vi "DAQX mod 1SDI v00.vi"(0 "resource name":refnum<k15>="PXI1Slot2", 1 "close (T)":bool=TRUE, 2 "Record Data":bool, 3 "numSamples":i32=-1, 4 "max time (s)":dbl=10.0 caption="max time", 5 "min sample rate":dbl=100000000.0, 6 "File location":path, 7 "error in":errorcluster, 8 "reference position":dbl=50.0, 9 "IIR filter specifications":T1={"Topology"=enum."Butterworth", "Type"=enum."Lowpass", "Order"=1, "Lower Fc"=100.0, "Upper Fc"=200.0, "PB Ripple"=1.0, "SB Attenuation"=60.0} {"PB Ripple" format="%0.2f"; "SB Attenuation" format="%0.2f"; "Lower Fc" format="%0.2p"; "Upper Fc" format="%0.2p"}, 10 "Type of\nmeasurement":u16, 11 "Name root":string, 12 "File Name":path=path "C:/Documents and Settings/QIM/My Documents/LabVIEW Data/111016-discord-gain9-seed40-3/ele-0000mV-d0150mV-g9-s40.lvm", 13 "channel parameters":T3(array[cluster])=[{"channel name"="0", "input impedance"=0, "maximum input frequency"=30000000.0, "vertical coupling"=1, "probe attenuation"=1.0, "vertical range"=2.0, "vertical offset"=0.0, "channel enabled"=TRUE}, {"channel name"="1", "input impedance"=0, "maximum input frequency"=30000000.0, "vertical coupling"=1, "probe attenuation"=1.0, "vertical range"=2.0, "vertical offset"=0.0, "channel enabled"=TRUE}] {"input impedance" items=["1 mega ohm"=0, "50 ohms"=2]; "vertical coupling" items=["AC", "DC", "Ground"]}, 14 "Shot noise start":bool, 15 "reset sn":bool) -> (16 "Signal 1":dbl[](graph), 17 "conditional variance":dbl, 18 "error out TDMS":errorcluster caption="error out", 19 "covariance":dbl, 20 "Variance 2 normalised to SNL":dbl(graph), 21 "Signal 2":dbl[](graph), 22 "Parameters values file":string, 23 "Variance 1 normalised to SNL":dbl(graph), 24 "actualSamples 0":i32, 26 "actualSamples 1":i32, 27 "error out":errorcluster caption="error out final")   [LabVIEW 2013]
doc: "Configures and acquires data from an NI-SCOPE high-speed digitizer.\n--------------------\n\nThis Express VI is configured as follows:\n\nDevice: PXI1Slot2 (PXI-5122)\nSample Rate (S/s): 100M\nRecord length: 2k\nAcquisition Mode: N Samples\nChannel 0\n - Range (V): 2\n - Offset (V): 0\n - Probe attenuation: 1\n - Coupling: \n - Input impedence: 1 \n - Bandwidth (Hz): 0\nChannel 1\n - Range (V): 2\n - Offset (V): 0\n - Probe attenuation: 1\n - Coupling: \n - Input impedence: 1 \n - Bandwidth (Hz): 0\nImmediate"
uses:
  <instrlib>/niScope/Controls/niScope vertical coupling.ctl
  <instrlib>/niScope/Controls/niScope timestamp type.ctl
  <vilib>/Analysis/5stat.llb/RMS (DBL).vi
  <vilib>/Analysis/baseanly.llb/Mean (DBL).vi
  <instrlib>/niScope/Acquire/Fetch/niScope Multi Fetch Binary 16.vi
  <instrlib>/niScope/Acquire/Fetch/niScope Multi Fetch WDT.vi
  <vilib>/measure/macond.llb/IIR Filter for N Chan.vi
  Global VIs/shotnoise.vi
  <instrlib>/niScope/Configure/Trigger/niScope Configure Trigger Immediate.vi
  <vilib>/measure/NI_MAPro.lvlib
  <vilib>/Analysis/NI_AALPro.lvlib
  <vilib>/Analysis/NI_AALBase.lvlib
panel:
  out "gain 1":dbl
  out "offset 1":dbl
  out "xIncrement 1":dbl
  out "relativeInitialX 1":dbl
  out "file location into parameter files":path
  out "size(s)":i32
  out "gain 0":dbl
  out "offset 0":dbl
  out "xIncrement 0":dbl
  out "relativeInitialX 0":dbl
  out "actual sample rate":dbl
  in  "Additional text":string
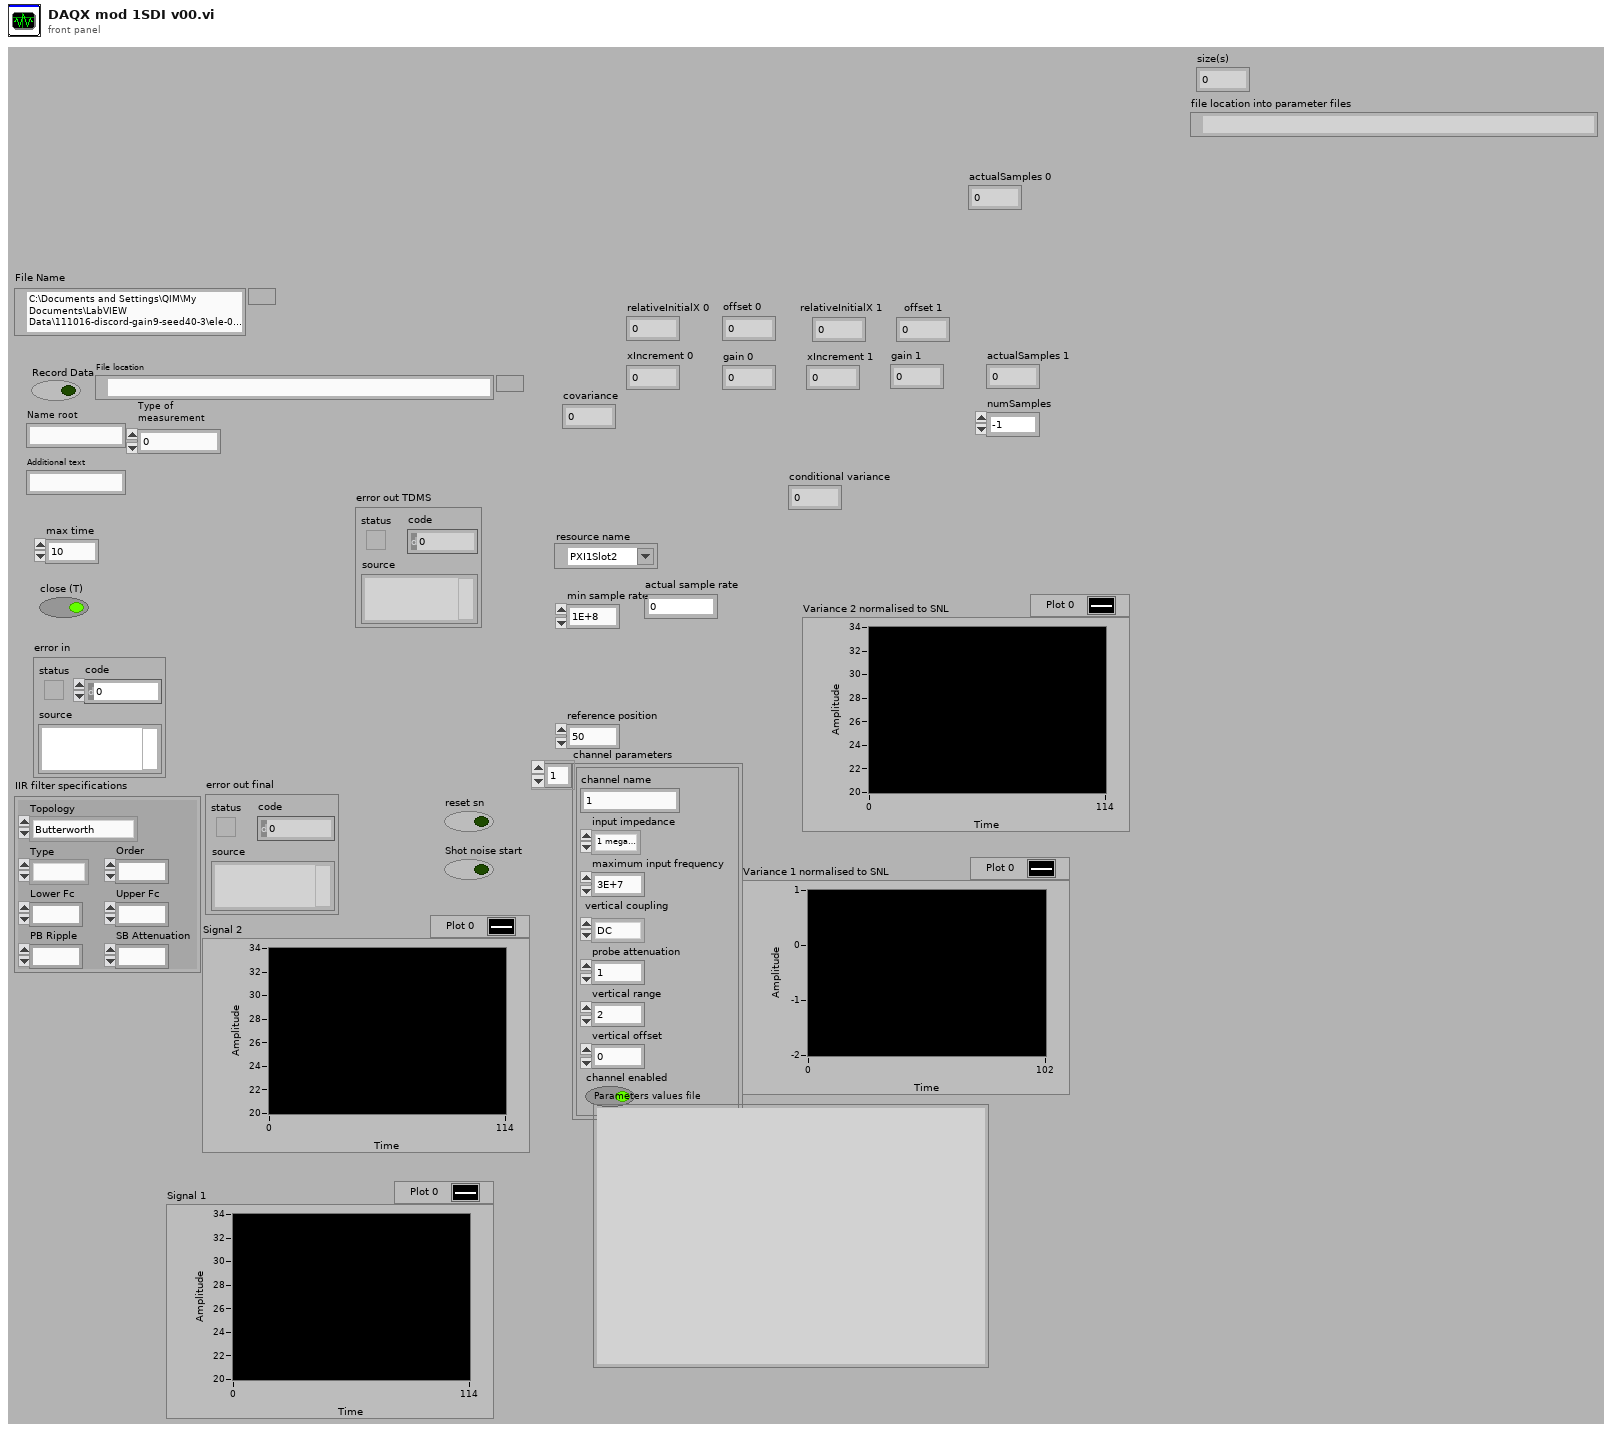
[diagram p1: front panel]
types:
  T1 = cluster{"Topology":enum16{"Off", "Butterworth", "Chebyshev", "Inverse Chebyshev", "Elliptic", "Bessel"}, "Type":enum16{"Lowpass", "Highpass", "Bandpass", "Bandstop"}, "Order":i32, "Lower Fc":dbl, "Upper Fc":dbl, "PB Ripple":dbl, "SB Attenuation":dbl}
  T2 = typedef "niScope vertical coupling.ctl" = i32
  T3 = cluster{"channel name":string, "input impedance":u32, "maximum input frequency":dbl, "vertical coupling":T2, "probe attenuation":dbl, "vertical range":dbl, "vertical offset":dbl, "channel enabled":bool}[]
  T4 = typedef "niScope timestamp type.ctl" = i32
  T5 = cluster{"actualSamples":i32, "absoluteInitialX":dbl, "relativeInitialX":dbl, "xIncrement":dbl, "offset":dbl, "gain":dbl, "reserved1":dbl, "reserved2":dbl}[]
  T6 = cluster{"actualSamples":i32, "absoluteInitialX":dbl, "relativeInitialX":dbl, "xIncrement":dbl, "offset":dbl, "gain":dbl, "reserved1":dbl, "reserved2":dbl}
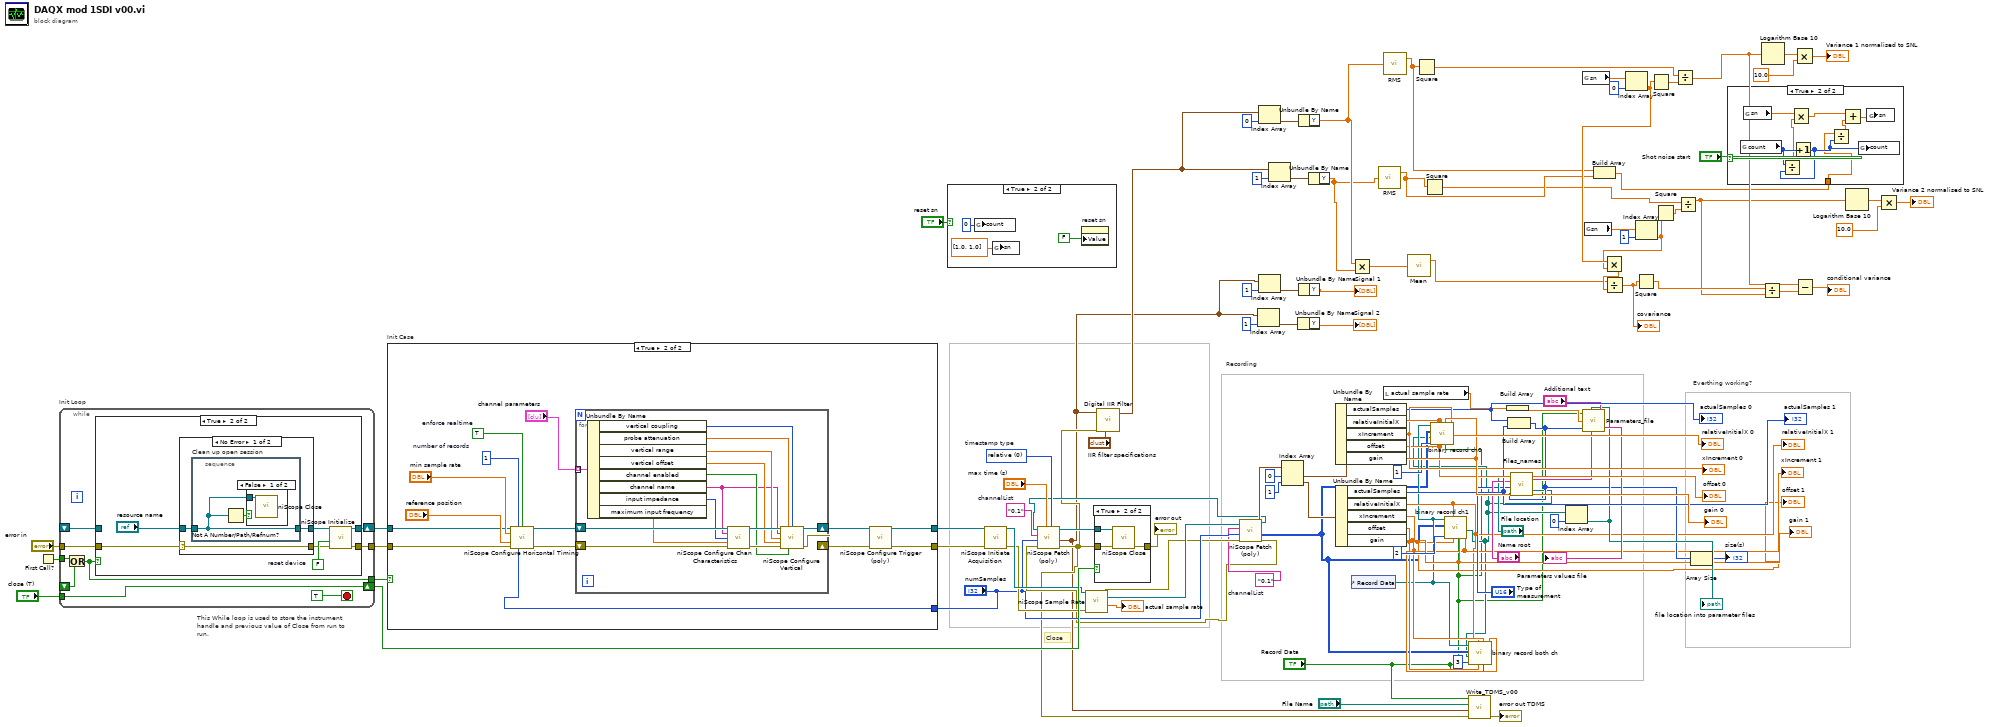
[diagram p0: block diagram]
diagram:
  w25 = "0,1"  # channelList
  w100 = T4 0 items=["relative", "absolute"]  # timestamp type
  w103 = "0,1"  # channelList
  # "Everthing working?"
  # "Recording"
  # "This While loop is used to store the instrument handle and previous value of Close from run to run."
  # "Close"
  n1 = First Call?() -> (First Call?: T/F=w99:bool)
  n2 = while "Init Loop" {
    tunnel: w99 -> [w114]
    shift-right: [w113] -> w95
    shift-left: _ -> [w110]
    tunnel: "close (T)" -> [w113]
    shift-right: [w112] -> w98
    shift-left: _ -> [w111]
    tunnel: [w108] -> w97
    tunnel: "error in" -> [w107]
    tunnel: [w106] -> w96
    stop <- TRUE ("stopInit") stop-if-true
    n3 = Or(x=w114, y=w110) -> (x .or. y?=w106:bool)
    n4 = case "Select_Init" shown="True" w106 {
      tunnel: [w116 w121] -> w112
      tunnel: w111 -> [w116 _]
      tunnel: [w115 w120] -> w108
      tunnel: w107 -> [w115 w119]
      frame False {
      }
      frame True {
        w122 = FALSE  # reset device
        n5 = case shown="No Error" w119 {
          selector: w119 -> [w124 w130]
          tunnel: [w126 w131] -> w123
          tunnel: "resource name" -> [w125 w131]
          tunnel: [w124 w130] -> w118
          frame No Error {
            n6 = stacked-sequence "Clean up open session" {
              tunnel: w125 -> [w127]
              tunnel: [w127] -> w126
              frame #0 {
                n7 = Not A Number/Path/Refnum?(number/path/refnum=w127) -> (NaN/Path/Refnum?=w128:bool)
                n8 = case shown="False" w128 {
                  tunnel: w127 -> [w129 _]
                  frame False {
                    n9 = call <instrlib>:"niScope Close.vi"("instrument handle"=w129) -> ()  [unwired: 1 in, 14 out]
                  }
                  frame True {
                  }
                }
              }
            }
          }
          frame Error {
          }
        }
        n10 = call <instrlib>:"niScope Initialize.vi"("resource name"=w123, "reset device"=w122, "error in"=w118) -> ("instrument handle"=w121:refnum<k15>, "error out"=w120:errorcluster)  [unwired: 2 in, 9 out]
      }
    }
  }
  n11 = case "Init Case" shown="True" w96 {
    tunnel: w97 -> [w132 w138]
    tunnel: [w132 w140] -> w102
    tunnel: [w133 w141] -> w101
    tunnel: w98 -> [w133 w139]
    tunnel: "numSamples" -> [_ w134]
    frame False {
    }
    frame True {
      w146 = 1  # number of records
      w147 = TRUE  # enforce realtime
      n12 = call <instrlib>:"niScope Configure Horizontal Timing.vi"("instrument handle"=w139, "number of records"=w146, "enforce realtime"=w147, "min sample rate"="min sample rate", "reference position"="reference position", "error in"=w138, "min record length"=w134) -> ("instrument handle out"=w142:refnum<k15>, "error out"=w143:errorcluster)  [unwired: 7 out]
      n13 = for {
        shift-right: [w150] -> w135
        shift-left: w143 -> [w162]
        shift-right: [w149] -> w136
        shift-left: w142 -> [w161]
        tunnel: "channel parameters" -> [w158] mode=indexing
        n14 = Unbundle By Name(w158) -> ("vertical coupling"=w155:T2, "probe attenuation"=w154:dbl, "vertical range"=w153:dbl, "vertical offset"=w152:dbl, "channel enabled"=w151:bool, "channel name"=w148:string, "input impedance"=w156:u32, "maximum input frequency"=w157:dbl)
        n15 = call <instrlib>:"niScope Configure Chan Characteristics.vi"("instrument handle"=w161, "channels"=w148, "input impedance"=w156, "maximum input frequency"=w157, "error in"=w162) -> ("instrument handle out"=w160:refnum<k15>, "error out"=w159:errorcluster)  [unwired: 9 out]
        n16 = call <instrlib>:"niScope Configure Vertical.vi"("instrument handle"=w160, "probe attenuation"=w154, "vertical coupling"=w155, "channels"=w148, "vertical range"=w153, "vertical offset"=w152, "error in"=w159, "channel enabled"=w151) -> ("instrument handle out"=w149:refnum<k15>, "error out"=w150:errorcluster)  [unwired: 6 out]
      }
      n17 = call-poly <instrlib>:"niScope Configure Trigger (poly).vi"("instrument handle"=w136, "error in"=w135) -> ("instrument handle out"=w141:refnum<k15>, "error out"=w140:errorcluster)  [unwired: 12 out]
    }
  }
  n18 = case shown="True" "reset sn" {
    frame False {
    }
    frame True {
      n19 = global write "shotnoise.vi" "count"(i64 0 ("count")) -> ()
      n20 = global write "shotnoise.vi" "sn"(dbl[] [1.0, 1.0] ("sn")) -> ()
      n21 = property on="reset sn" class="Bool (strict)"("Value"=FALSE ("reset sn")) -> ()  [unwired: 2 in, 2 out]
    }
  }
  n22 = call <instrlib>:"niScope Initiate Acquisition.vi"("instrument handle"=w101, "error in"=w102) -> ("instrument handle out"=w84:refnum<k15>, "error out"=w83:errorcluster)  [unwired: 12 out]
  n23 = call <instrlib>:"niScope Sample Rate.vi"("instrument handle"=w84, "error in"=w83) -> ("instrument handle out"=w52:refnum<k15>, "actual sample rate"=→"actual sample rate":dbl, "error out"=w51:errorcluster)  [unwired: 11 out]
  n24 = call-poly <instrlib>:"niScope Fetch (poly).vi"("error in"=w51, "numSamples"="numSamples", "channels"=w25, "instrument handle"=w52) -> ("error out"=w18:errorcluster, "wfm"=w14:i16[][], "wfm info"=w50:T5, "instrument handle out"=w19:refnum<k15>)  [unwired: 1 in, 3 out]
  n25 = call-poly <instrlib>:"niScope Fetch (poly).vi"("timestamp Type"=w100, "timeout"="max time (s)", "error in"=w18, "numSamples"="numSamples", "channels"=w103, "instrument handle"=w19) -> ("error out"=w10:errorcluster, "wfm"=w1:waveform(dbl)[], "instrument handle out"=w82:refnum<k15>)  [unwired: 3 out]
  n26 = case shown="True" w95 {
    tunnel: w10 -> [w166 w169]
    tunnel: [w166 w168] -> w105
    tunnel: w82 -> [_ w167]
    frame False {
    }
    frame True {
      n27 = call <instrlib>:"niScope Close.vi"("instrument handle"=w167, "error in"=w169) -> ("error out"=w168:errorcluster)  [unwired: 13 out]
    }
  }
  "error out" <- w105
  n28 = call-poly <vilib>:"Digital IIR Filter.vi"("IIR filter specifications"="IIR filter specifications", "error in (no error)"=w10, "signal(s) in"=w1) -> ("signal(s) out"=w71:waveform(dbl)[])  [unwired: 3 in, 5 out]
  n29 = Index Array(array=w1, index=1) -> (element=w6:waveform(dbl))
  n30 = Index Array(array=w71, index=0) -> (element=w78:waveform(dbl))
  n31 = Index Array(array=w1, index=1) -> (element=w3:waveform(dbl))
  n32 = Index Array(array=w71, index=1) -> (element=w73:waveform(dbl))
  n33 = Index Array(array=w50, index #1=0 ("index"), index #2=1 ("index")) -> (element #1=w47:T6, element #2=w46:T6)
  n34 = Unbundle By Name(w6) -> ("Y"=→"Signal 2":dbl[])
  n35 = Unbundle By Name(w78) -> ("Y"=w17:dbl[])
  n36 = Unbundle By Name(w3) -> ("Y"=→"Signal 1":dbl[])
  n37 = Unbundle By Name(w73) -> ("Y"=w8:dbl[])
  n38 = Unbundle By Name(w47) -> ("actualSamples"=w39:i32, "relativeInitialX"=w45:dbl, "xIncrement"=w43:dbl, "offset"=w42:dbl, "gain"=w44:dbl)
  "actualSamples 0" <- w39
  "relativeInitialX 0" <- w45
  "xIncrement 0" <- w43
  "offset 0" <- w42
  "gain 0" <- w44
  n39 = Unbundle By Name(w46) -> ("actualSamples"=w38:i32, "relativeInitialX"=w22:dbl, "xIncrement"=w23:dbl, "offset"=w21:dbl, "gain"=w24:dbl)
  "actualSamples 1" <- w38
  "relativeInitialX 1" <- w22
  "xIncrement 1" <- w23
  "offset 1" <- w21
  "gain 1" <- w24
  n40 = Multiply(x=w17, y=w8) -> (x*y=w54:dbl[])
  n41 = control-ref of="Record Data"() -> (w15:refnum<vi>)
  n42 = call-poly <vilib>:"RMS.vi"("X"=w8) -> ("rms value"=w56:dbl)  [unwired: 1 out]
  n43 = local read "actual sample rate"() -> (w29:dbl)
  n44 = call-poly <vilib>:"RMS.vi"("X"=w17) -> ("rms value"=w58:dbl)  [unwired: 1 out]
  n45 = call-poly <vilib>:"Mean.vi"("X"=w54) -> ("mean"=w53:dbl)  [unwired: 1 out]
  n46 = Square(x=w58) -> (x^2=w57:dbl)
  n47 = Square(x=w56) -> (x^2=w55:dbl)
  n48 = call "Write_TDMS_v00.vi"("error in"=w10, "Waveform"=w1, "File Name"="File Name", "Record Data"="Record Data") -> ("error out"=→"error out TDMS":errorcluster)  [unwired: 7 in]
  n49 = Build Array(w29) -> (w28:dbl[])
  n50 = Build Array(w39, w38) -> (w27:i32[])
  n51 = call "Files_names.vi"("actualSamples\narray"=w27, "Type of\nmeasurement"="Type of\nmeasurement", "Name root"="Name root", "File location"="File location") -> ("Files path array"=w13:path[], "Files name array"=w34:string[])
  n52 = call "binary record ch0.vi"("xIncrement"=w43, "Record"="Record Data", "gain"=w44, "offset"=w42, "relativeInitialX"=w45, "Index files\npath array"=1 ("Index files\npath array"), "Files path array"=w13, "wfm"=w14, "reference"=w15) -> ()  [unwired: 3 out]
  n53 = call "binary record ch1.vi"("xIncrement"=w23, "Record"="Record Data", "gain"=w24, "offset"=w21, "relativeInitialX"=w22, "Index files\npath array"=2 ("Index files\npath array"), "Files path array"=w13, "wfm"=w14, "reference"=w15) -> ()  [unwired: 3 out]
  n54 = call "binary record both ch.vi"("xIncrement"=w23, "Record"="Record Data", "gain"=w24, "offset"=w21, "relativeInitialX"=w22, "Index files\npath array"=3 ("Index files\npath array"), "Files path array"=w13, "wfm"=w14, "reference"=w15) -> ()  [unwired: 3 out]
  n55 = Index Array(array=w13, index=0) -> (element=w31:path)
  "file location into parameter files" <- w31
  n56 = global read "shotnoise.vi" "sn"() -> (w76:dbl[])
  n57 = call "Parameters_file.vi"("Record"="Record Data", "File location"=w31, "actual sample rate array"=w28, "actualSamples array"=w27, "Files name array"=w34, "Additional text"="Additional text") -> ("Full text"=→"Parameters values file":string)
  n58 = global read "shotnoise.vi" "sn"() -> (w75:dbl[])
  n59 = Build Array(w58, w56) -> (w59:dbl[])
  n60 = Index Array(array=w76, index=0) -> (element=w63:dbl)
  n61 = Index Array(array=w75, index=1) -> (element=w62:dbl)
  n62 = Multiply(x=w63, y=w62) -> (x*y=w61:dbl)
  n63 = Divide(x=w53, y=w61) -> (x/y=w16:dbl)
  "covariance" <- w16
  n64 = Square(x=w16) -> (x^2=w69:dbl)
  n65 = Square(x=w63) -> (x^2=w66:dbl)
  n66 = Square(x=w62) -> (x^2=w64:dbl)
  n67 = Divide(x=w57, y=w66) -> (x/y=w65:dbl)
  n68 = Divide(x=w55, y=w64) -> (x/y=w60:dbl)
  n69 = Array Size(array=w27) -> (size(s)=→"size(s)":i32)
  n70 = case shown="True" "Shot noise start" {
    tunnel: w59 -> [_ w171]
    frame False {
    }
    frame True {
      n71 = global read "shotnoise.vi" "count"() -> (w176:i64)
      n72 = global read "shotnoise.vi" "sn"() -> (w175:dbl[])
      n73 = Increment(x=w176) -> (x+1=w172:i64)
      n74 = Divide(x=w176, y=w172) -> (x/y=w174:dbl)
      n75 = Multiply(x=w175, y=w174) -> (x*y=w173:dbl[])
      n76 = Divide(x=w171, y=w172) -> (x/y=w170:dbl[])
      n77 = Add(x=w173, y=w170) -> (x+y=w177:dbl[])
      n78 = global write "shotnoise.vi" "count"(w172) -> ()
      n79 = global write "shotnoise.vi" "sn"(w177) -> ()
    }
  }
  n80 = Divide(x=w69, y=w60) -> (x/y=w68:dbl)
  n81 = Logarithm Base 10(1:w65) -> (0:w91:dbl)
  n82 = Multiply(x=w91, y=10.0) -> (x*y=→"Variance 1 normalised to SNL":dbl)
  n83 = Subtract(x=w65, y=w68) -> (x-y=→"conditional variance":dbl)
  n84 = Logarithm Base 10(1:w60) -> (0:w88:dbl)
  n85 = Multiply(x=w88, y=10.0) -> (x*y=→"Variance 2 normalised to SNL":dbl)
